vi "labview_pid_test.vi"() -> ()   [LabVIEW 2019]
panel:
  out "Is the PID fnished?":bool[](array[boolean])
  out "I val":i32
  out "return value 2":dbl[](array[numeric])
  in  "stop":bool
  out "return value 1":dbl[](array[numeric])
  out "Iteration counter":i32
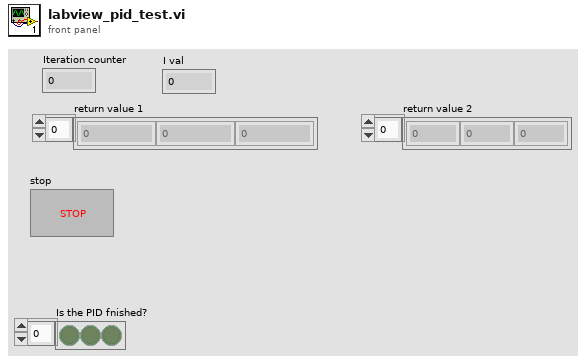
[diagram p1: front panel]
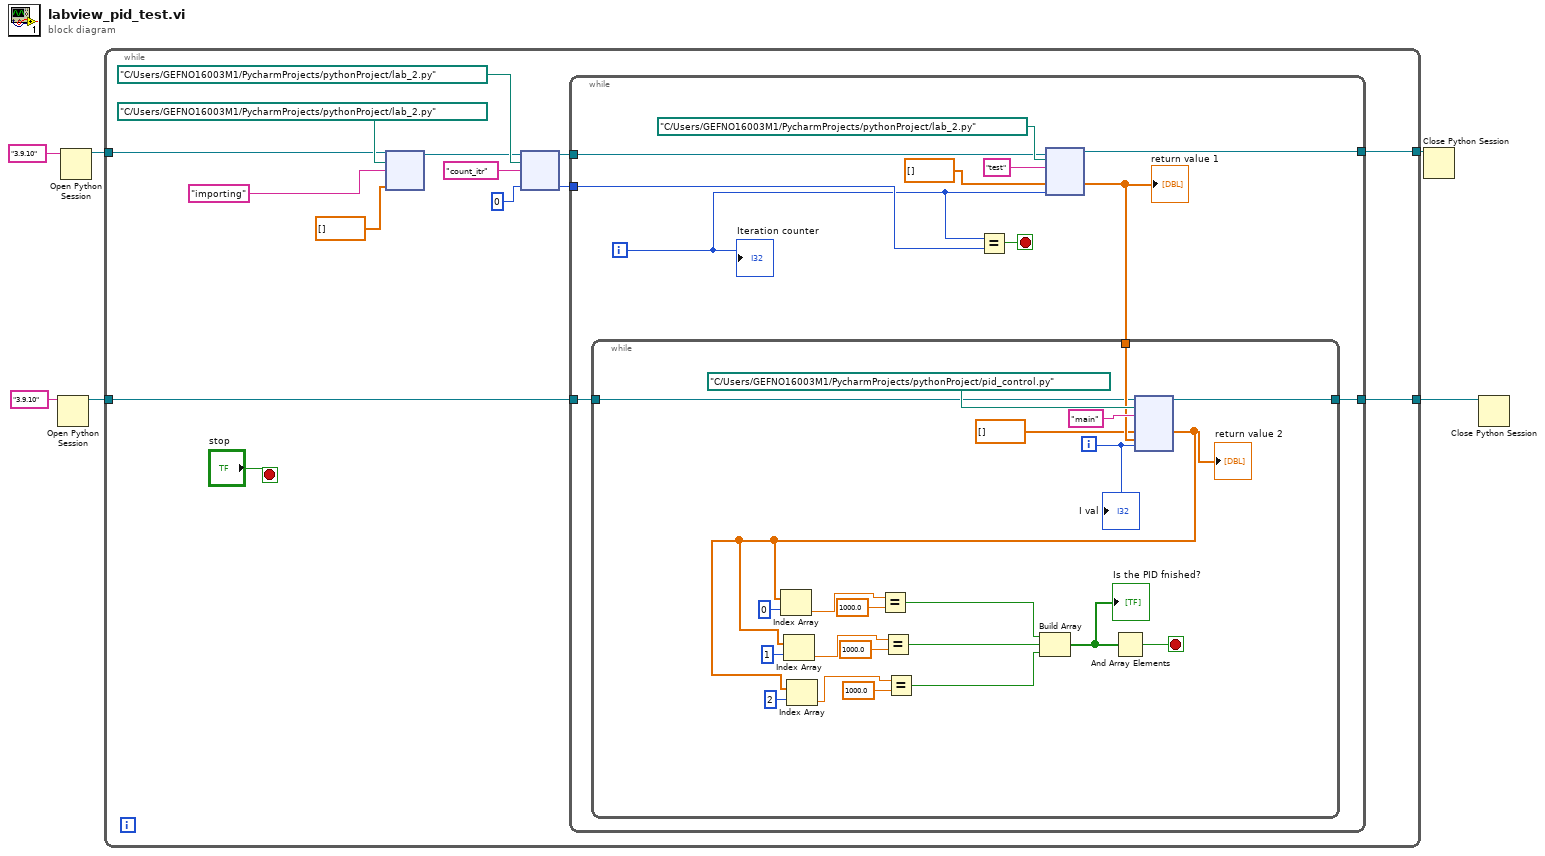
[diagram p0: block diagram]
diagram:
  n1 = Open Python Session(python version="3.9.10" ("Python version")) -> (session out=w2:refnum<k35>)  [unwired: 2 in, 1 out]
  n2 = Open Python Session(python version="3.9.10" ("Python version")) -> (session out=w5:refnum<k35>)  [unwired: 2 in, 1 out]
  n3 = while {
    tunnel: w5 -> [w10]
    tunnel: [w9] -> w4
    tunnel: w2 -> [w8]
    tunnel: [w7] -> w1
    stop <- "stop" stop-if-true
    n4 = node(w10, path "C:/Users/GEFNO16003M1/PycharmProjects/pythonProject/lab_2.py" ("module path"), "importing" ("function name"), dbl[] []) -> (w15:refnum<k35>)  [unwired: 2 in, 3 out]
    n5 = node(w15, path "C:/Users/GEFNO16003M1/PycharmProjects/pythonProject/lab_2.py" ("module path"), "count_itr" ("function name"), 0) -> (w14:refnum<k35>, w12:i32)  [unwired: 1 in, 3 out]
    n6 = while {
      tunnel: [w25] -> w9
      tunnel: w14 -> [w28]
      tunnel: w12 -> [w26]
      tunnel: w8 -> [w22]
      tunnel: [w21] -> w7
      i -> [w23]
      stop <- w29 stop-if-true
      n7 = Equal?(x=w23, y=w26) -> (x = y?=w29:bool)
      n8 = node(w28, path "C:/Users/GEFNO16003M1/PycharmProjects/pythonProject/lab_2.py" ("module path"), "test" ("function name"), dbl[] [], w23) -> (w25:refnum<k35>, w24:dbl[])  [unwired: 2 in, 3 out]
      "return value 1" <- w24
      n9 = while {
        tunnel: w24 -> [w51]
        tunnel: w22 -> [w49]
        tunnel: [w48] -> w21
        i -> [w47]
        stop <- w33 stop-if-true
        n10 = node(w49, path "C:/Users/GEFNO16003M1/PycharmProjects/pythonProject/pid_control.py" ("module path"), "main" ("function name"), dbl[] [], w51, w47) -> (w48:refnum<k35>, w37:dbl[])  [unwired: 3 in, 3 out]
        "return value 2" <- w37
        n11 = Index Array(array=w37, index=0) -> (element=w40:dbl)
        n12 = Index Array(array=w37, index=1) -> (element=w39:dbl)
        n13 = Index Array(array=w37, index=2) -> (element=w38:dbl)
        n14 = Equal?(x=w40, y=1000.0) -> (x = y?=w36:bool)
        n15 = Equal?(x=w39, y=1000.0) -> (x = y?=w35:bool)
        n16 = Equal?(x=w38, y=1000.0) -> (x = y?=w34:bool)
        n17 = Build Array(w36, w35, w34) -> (w32:bool[])
        "Is the PID fnished?" <- w32
        n18 = And Array Elements(Boolean array=w32) -> (logical AND=w33:bool)
        "I val" <- w47
      }
      "Iteration counter" <- w23
    }
  }
  n19 = Close Python Session(session in=w4) -> ()  [unwired: 1 in, 1 out]
  n20 = Close Python Session(session in=w1) -> ()  [unwired: 1 in, 1 out]
